vi "CheckScreenShot (SubVI).vi"(11 "VI reference":refnum<vi>) -> ()   [LabVIEW 2013]
uses:
  <vilib>/picture/picture.llb/Draw True-Color Pixmap.vi
panel:
  out "ScreenShot":picture
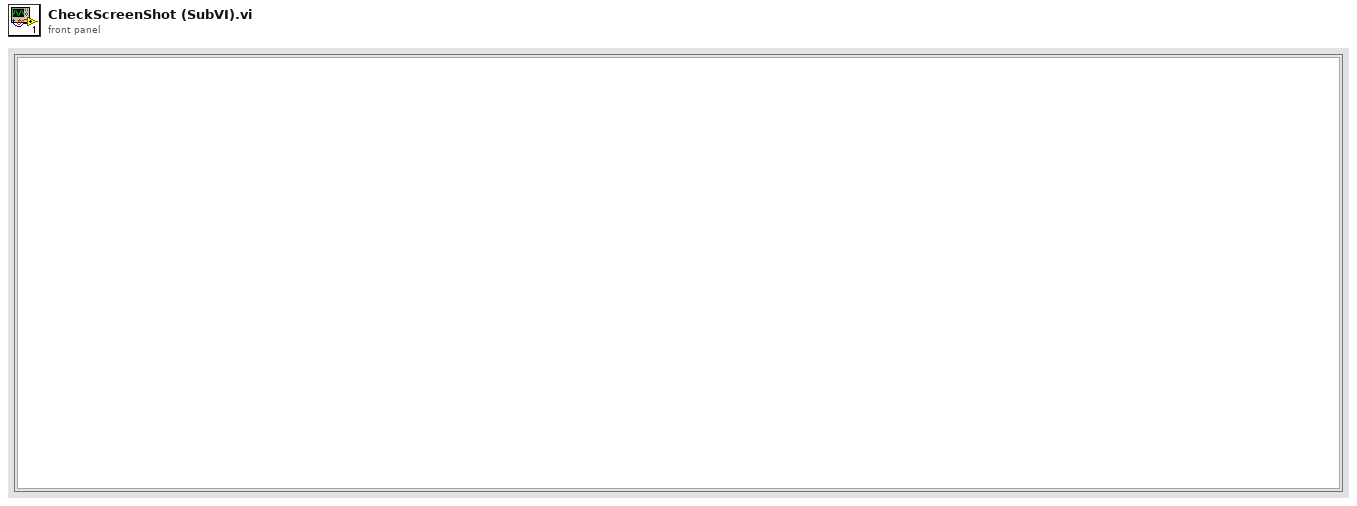
[diagram p1: front panel]
types:
  T1 = typedef "imagedata.ctl" = cluster{"image type":i32, "image depth":i32, "image":u8[], "mask":u8[], "colors":u32[], "Rectangle":cluster{"left":i16, "top":i16, "right":i16, "bottom":i16}}
  T2 = typedef "LVRectTypeDef.ctl" = cluster{"Left":i16, "Top":i16, "Right":i16, "Bottom":i16}
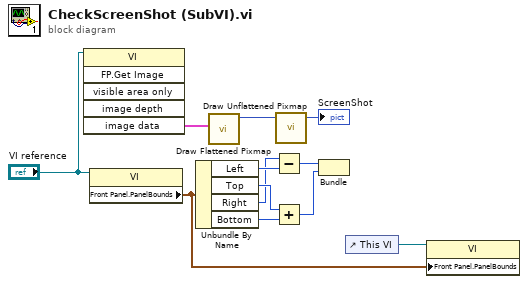
[diagram p0: block diagram]
diagram:
  n1 = invoke class="VI" method="FP.Get Image"(reference="VI reference") -> ("image data"=w11:T1)  [unwired: 5 in, 5 out]
  n2 = property class="VI"(reference="VI reference") -> ("Front Panel.PanelBounds"=w1:T2)  [unwired: 1 in, 2 out]
  n3 = Unbundle By Name(w1) -> ("Left"=w4:i16, "Top"=w8:i16, "Right"=w3:i16, "Bottom"=w7:i16)
  n4 = call <vilib>:"Draw Flattened Pixmap.vi"("image data"=w11) -> ("new picture"=w12:picture)  [unwired: 8 in]
  n5 = Subtract(x=w3, y=w4) -> (x-y=w6:i16)
  n6 = Add(x=w8, y=w7) -> (x+y=w5:i16)
  n7 = call-poly <vilib>:"Draw Unflattened Pixmap.vi"("picture"=w12) -> ("new picture"=→"ScreenShot":picture)  [unwired: 8 in]
  n8 = Bundle(w6, w5) -> ()  [unwired: 1 in, 1 out]
  n9 = control-ref of="This VI"() -> (w2:refnum<vi>)
  n10 = property class="VI"(reference=w2, "Front Panel.PanelBounds"=w1) -> ()  [unwired: 1 in, 2 out]
